vi "send trigger.vi"() -> ()   [LabVIEW 2011]
uses:
  <vilib>/DAQmx/write.llb/DAQmx Write (Digital 1D U8 1Chan NSamp).vi
  <vilib>/DAQmx/miscellaneous.llb/DAQmx Fill In Error Info.vi
panel:
  in  "set id":bool
  in  "trigger id":u8
  in  "send":bool
  in  "stop":bool
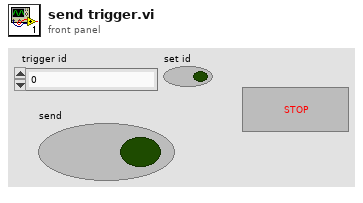
[diagram p1: front panel]
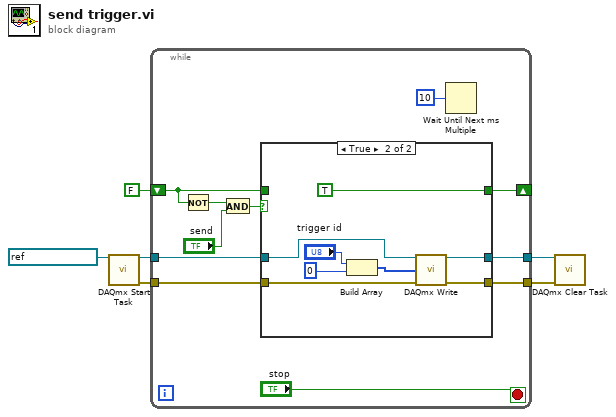
[diagram p0: block diagram]
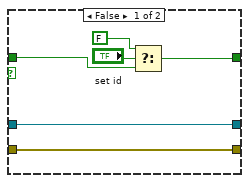
[diagram p2: hidden frame]
diagram:
  n1 = call <vilib>:"DAQmx Start Task.vi"("task/channels in"=refnum<k21> "TriggerDPort" ("DAQmx Task Name")) -> ("task out"=w5:refnum<k21>, "error out"=w2:errorcluster)  [unwired: 13 in]
  n2 = while {
    tunnel: w5 -> [w17]
    tunnel: [w15] -> w4
    tunnel: [w14] -> w3
    tunnel: w2 -> [w13]
    shift-right: [w12] -> _
    shift-left: FALSE -> [w8]
    stop <- "stop" stop-if-true
    n3 = Not(x=w8) -> (.not. x?=w9:bool)
    n4 = And(x=w9, y="send") -> (x .and. y?=w11:bool)
    n5 = case shown="True" w11 {
      tunnel: w17 -> [w23 w31]
      tunnel: [w23 w28] -> w15
      tunnel: [w22 w27] -> w14
      tunnel: w13 -> [w22 w30]
      tunnel: [w19 TRUE] -> w12
      tunnel: w8 -> [w20 _]
      frame False {
        n6 = Select(t=FALSE, s="set id", f=w20) -> (s? t:f=w19:bool)
      }
      frame True {
        n7 = Build Array("trigger id", u8 0 ("element")) -> (w25:u8[])
        n8 = call-poly <vilib>:"DAQmx Write.vi"("task/channels in"=w31, "data"=w25, "error in"=w30) -> ("task out"=w28:refnum<k21>, "error out"=w27:errorcluster)  [unwired: 10 in, 1 out]
      }
    }
    n9 = Wait Until Next ms Multiple(millisecond multiple=u32 10) -> ()  [unwired: 1 out]
  }
  n10 = call <vilib>:"DAQmx Clear Task.vi"("task in"=w4, "error in"=w3) -> ()  [unwired: 13 in, 1 out]
